vi "CCM-Read Connection Table (by device).vi"(0 "Path In":path, 2 "IO Type":T1, 7 "Channels By Device":cluster{"Out":string[], "In":string[]}[](array[cluster]), 11 "error in (no error)":errorcluster) -> (4 "Path Out":path, 8 "Endpoints by Device":cluster{"Endpoints (by channel)":string[]}[](array[cluster]), 15 "error out":errorcluster)   [LabVIEW 2015]
uses:
  Type Defs/CM-IO Type.ctl
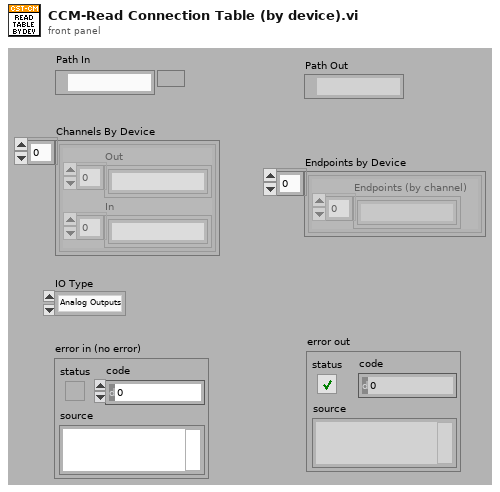
[diagram p1: front panel]
types:
  T1 = typedef "CM-IO Type.ctl" = enum16{"Analog Outputs", "Analog Inputs", "Digital Outputs", "Digital Inputs"}
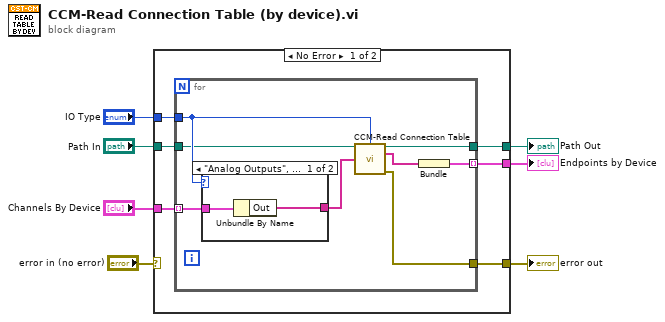
[diagram p0: block diagram]
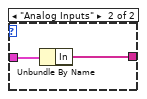
[diagram p2: hidden frame]
diagram:
  n1 = case shown="No Error" "error in (no error)" {
    selector: "error in (no error)" -> [_ w27]
    tunnel: "IO Type" -> [w13 _]
    tunnel: "Channels By Device" -> [w12 _]
    tunnel: "Path In" -> [w11 w26]
    tunnel: [w9 w27] -> w3
    tunnel: [w10 w26] -> w2
    tunnel: [w8 _] -> w1
    frame No Error {
      n2 = for {
        tunnel: w13 -> [w19]
        tunnel: w12 -> [w21] mode=indexing
        tunnel: w11 -> [w18]
        tunnel: [w17] -> w10
        tunnel: [w15] -> w8 mode=indexing
        tunnel: [w14] -> w9
        n3 = case shown="\"Analog Outputs\", Default" w19 {
          tunnel: w21 -> [w23 w25]
          tunnel: [w22 w24] -> w20
          frame "Analog Outputs", Default {
            n4 = Unbundle By Name(w23) -> ("Out"=w22:string[])
          }
          frame "Analog Inputs" {
            n5 = Unbundle By Name(w25) -> ("In"=w24:string[])
          }
        }
        n6 = call "CCM-Read Connection Table.vi"("Path In"=w18, "Type"=w19, "IOChannels"=w20) -> ("Path Out"=w17:path, "Endpoints (by channel)"=w16:string[], "error out"=w14:errorcluster)  [unwired: 9 in, 1 out]
        n7 = Bundle("Endpoints (by channel)"=w16) -> (w15:cluster{"Endpoints (by channel)":string[]})  [unwired: 1 in]
      }
    }
    frame Error {
    }
  }
  "error out" <- w3
  "Path Out" <- w2
  "Endpoints by Device" <- w1
